vi "Assert Not Equal Value_Variant.vi"(4 "Execution time (s)":dbl=-1.0, 5 "Assert Only? (F)":bool, 6 "error code (1)":i32=1, 7 "Label":string, 8 "error in (no error)":errorcluster, 9 "Register with caller test (F)":bool, 10 "Y":variant, 11 "X":variant) -> (0 "error out":errorcluster, 2 "Properties.Assert":refnum<class "Properties.Assert.lvclass">)   [LabVIEW 2013, in "Caraya.lvlib" / "Assert.lvclass"]
doc: "Generates an error if the input condition is not met.\n\nThis method compares the value of the inputs, irrespective of the type representation.\nAsserts TRUE if input values are not equal.\nAsserts FALSE otherwise.\n\nex 1: Two integer inputs of different value will assert TRUE, whether or not they are of same type representation.\n\nex 2: Two integer inputs of equal value but of different type representation (U8 and I32) will assert FALSE."
uses:
  Assert.lvclass
  Properties.Assert/Properties.Assert.lvclass
  Properties/Properties.lvclass
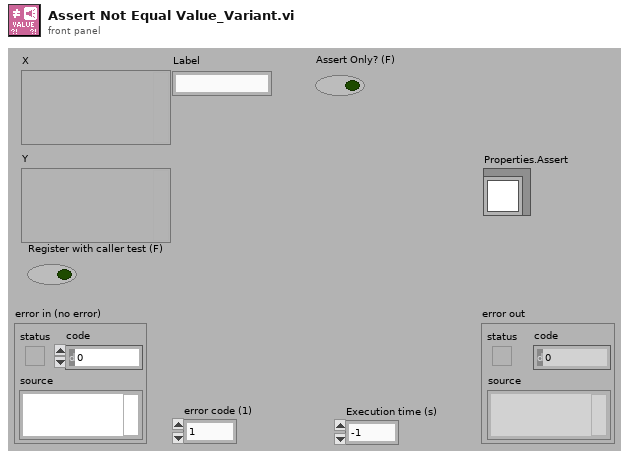
[diagram p1: front panel]
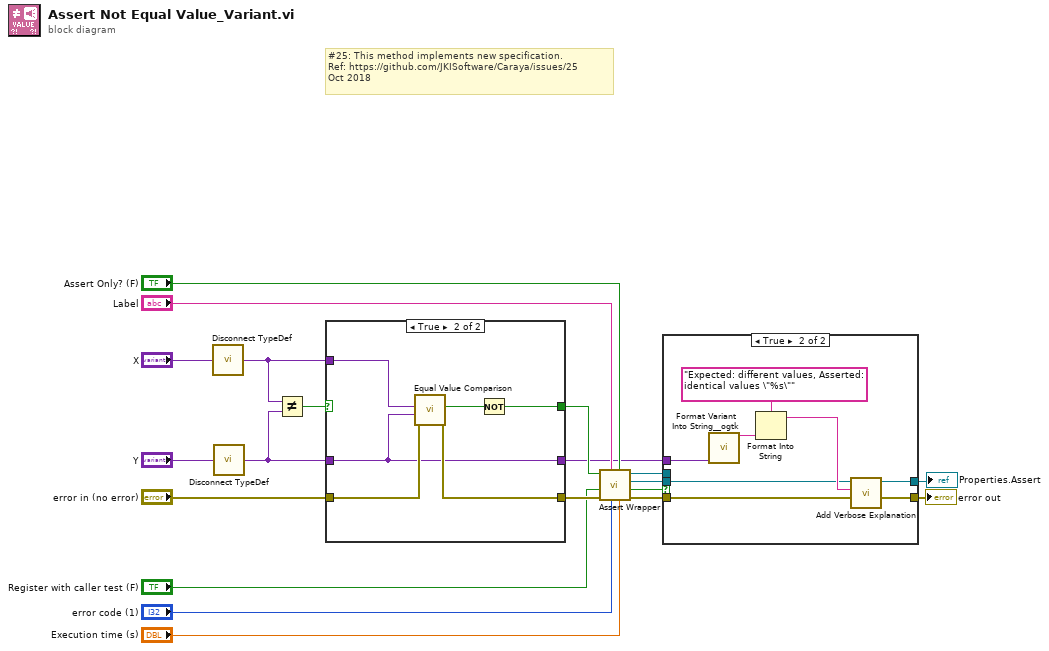
[diagram p0: block diagram]
diagram:
  # "#25: This method implements new specification.\nRef: https://github.com/JKISoftware/Caraya/issues/25\nOct 2018"
  n1 = call "Disconnect TypeDef.vi"("Variant"="X") -> ("Variant Out"=w13:variant)
  n2 = call "Disconnect TypeDef.vi"("Variant"="Y") -> ("Variant Out"=w11:variant)
  n3 = Not Equal?(x=w13, y=w11) -> (x != y?=w17:bool)
  n4 = case shown="True" w17 {
    selector: w17 -> [w23 _]
    tunnel: w13 -> [_ w25]
    tunnel: [w23 w28] -> w16
    tunnel: w11 -> [w21 w24]
    tunnel: "error in (no error)" -> [w22 w26]
    tunnel: [w22 w27] -> w15
    tunnel: [w21 w24] -> w7
    frame False {
      # "If they are equal, it means the Values are equal.\nAsserts FALSE"
    }
    frame True {
      n5 = call "Equal Value Comparison.vi"("error in (no error)"=w26, "Y"=w24, "X"=w25) -> ("error out"=w27:errorcluster, "Equal Values?"=w29:bool)  [unwired: 6 in, 1 out]
      n6 = Not(x=w29) -> (.not. x?=w28:bool)
    }
  }
  n7 = call "Assert Wrapper.vi"("Execution time (s)"="Execution time (s)", "Assert Only? (F)"="Assert Only? (F)", "error code (1)"="error code (1)", "Label"="Label", "error in (no error)"=w15, "Register with caller test (F)"="Register with caller test (F)", "Assert?"=w16) -> ("error out"=w5:errorcluster, "Verbose"=w6:bool, "Properties.Assert"=w2:refnum<class "Properties.Assert.lvclass">, "Assert out"=w3:refnum<class "Assert.lvclass">)  [unwired: 1 in]
  n8 = case shown="True" w6 {
    tunnel: [w31 w34] -> w9
    tunnel: w3 -> [_ _]
    tunnel: w5 -> [w31 w36]
    tunnel: w7 -> [_ w39]
    tunnel: w2 -> [w30 w33]
    tunnel: [w30 w32] -> w1
    frame False {
    }
    frame True {
      n9 = call <userlib>:"Format Variant Into String__ogtk.vi"("Variant"=w39) -> ("Output String"=w38:string)  [unwired: 13 in, 1 out]
      n10 = Format Into String(format string="Expected: different values, Asserted: identical values \"%s\"" ("t"), w38) -> (resulting string=w35:string)  [unwired: 2 in, 1 out]
      n11 = call "Add Verbose Explanation.vi"("error in (no error)"=w36, "Verbose Explanation"=w35, "Properties"=w33) -> ("error out"=w34:errorcluster, "Properties"=w32:refnum<class "Properties.Assert.lvclass">)  [unwired: 7 in]
    }
  }
  "error out" <- w9
  "Properties.Assert" <- w1
